vi "Allocate Device Handle.vi"(8 "Error In":errorcluster) -> (0 "Error Out":errorcluster, 3 "Device Handle":u64)   [LabVIEW 2011, in "LVH-Adept.lvlib" / "DMGR.lvlib"]
uses:
  DMGR.lvlib
  Resources/LVH-Adept Helper/LVH-Adept Helper/Debug/LVH-Adept Helper.dll
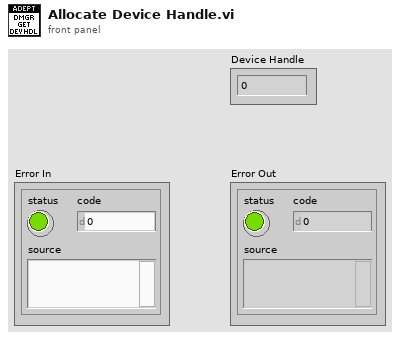
[diagram p1: front panel]
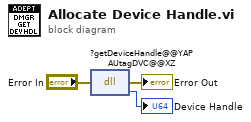
[diagram p0: block diagram]
diagram:
  n1 = dll-call lib="C:/github/labviewhacker/LVH-Adept/LabVIEW/vi.lib/LabVIEW Hacker/Adept/Private/Resources/LVH-Adept Helper/LVH-Adept Helper/Debug/LVH-Adept Helper.dll" fn="?getDeviceHandle@@YAPAUtagDVC@@XZ"(error in="Error In") -> (error out=→"Error Out":errorcluster, "devHandlePtr"=→"Device Handle":u64)  [unwired: 2 in, 1 out]
